vi "BlockDiagram_CreateTerminals.vi"(6 "error in":errorcluster, 9 "PythonConverter_BD in":refnum<class "PyConvBD.lvclass">) -> (0 "error out":errorcluster, 3 "PythonConverter_BD out":refnum<class "PyConvBD.lvclass">, 4 "create_terminals":string)   [LabVIEW 2014, in "PyConvBD.lvclass"]
uses:
  PyConvBD.lvclass
  Parsing/ClassTypeTD.ctl
  PyConvBD.lvclass/PyConvBD.ctl
  VI Interpreter/Classes/ControlTerminal/ControlTerminal.lvclass
  VI Interpreter/Classes/TopLevelDiagram/TopLevelDiagram.lvclass
  Parsing/Python Functions.lvlib
  VI Interpreter/Classes/VI Interpreter/VI Interpreter.lvclass
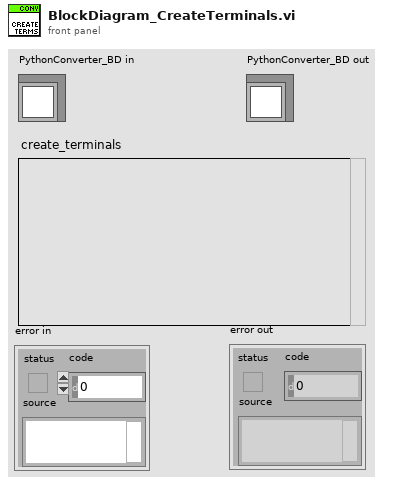
[diagram p1: front panel]
types:
  T1 = typedef "Python Functions.lvlib/ClassTypeTD.ctl" = enum16{"class", "function"}
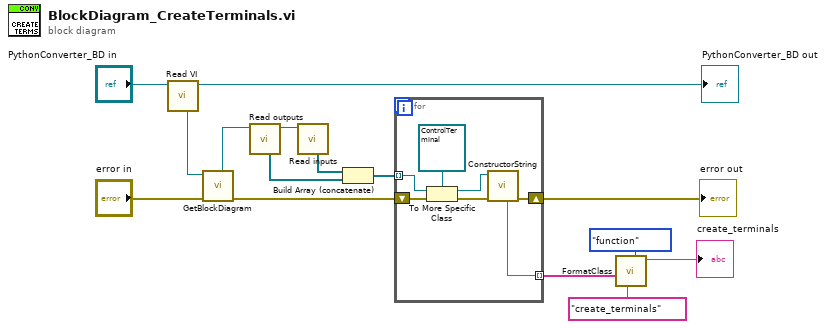
[diagram p0: block diagram]
diagram:
  n1 = call "Read VI.vi"("PythonConverter_BD in"="PythonConverter_BD in") -> ("PythonConverter_BD out"=→"PythonConverter_BD out":refnum<class "PyConvBD.lvclass">, "VI Interpreter"=w11:refnum<class "VI Interpreter.lvclass">)  [unwired: 7 in]
  n2 = call "GetBlockDiagram.vi"("error in"="error in", "VI Interpreter in"=w11) -> ("error out"=w12:errorcluster, "TopLevelDiagram"=w4:refnum<class "TopLevelDiagram.lvclass">)  [unwired: 5 in, 1 out]
  n3 = call-dynamic "Read outputs.vi"("Diagram in"=w4) -> ("Diagram out"=w5:refnum<class "TopLevelDiagram.lvclass">, "outputs"=w2:refnum<class "Terminal.lvclass">[])  [unwired: 7 in]
  n4 = call-dynamic "Read inputs.vi"("Diagram in"=w5) -> ("inputs"=w3:refnum<class "Terminal.lvclass">[])  [unwired: 7 in, 1 out]
  n5 = Build Array (concatenate)(w3, w2) -> (w1:refnum<class "Terminal.lvclass">[])
  n6 = for {
    tunnel: w1 -> [w20] mode=indexing
    shift-right: [w16] -> w7
    shift-left: w12 -> [w22]
    tunnel: [w17] -> w13 mode=indexing
    n7 = To More Specific Class(target class=refnum<class "ControlTerminal.lvclass"> refnum ("Control Terminal in"), reference=w20, error in=w22) -> (specific class reference=w18:refnum<class "ControlTerminal.lvclass">, error out=w19:errorcluster)
    n8 = call "ConstructorString.vi"("error in"=w19, "Control Terminal in"=w18) -> ("error out"=w16:errorcluster, "constructor"=w17:string)  [unwired: 5 in, 1 out]
  }
  "error out" <- w7
  n9 = call "FormatClass.vi"("type"=ClassTypeTD."function", "name"="create_terminals", "body"=w13) -> ("python"=→"create_terminals":string)  [unwired: 8 in]
